vi "Get Total Plays.vi"(0 "File Directory":path, 11 "error in (no error)":errorcluster) -> (4 "Total Plays":i32, 15 "error out":errorcluster)   [LabVIEW 2014]
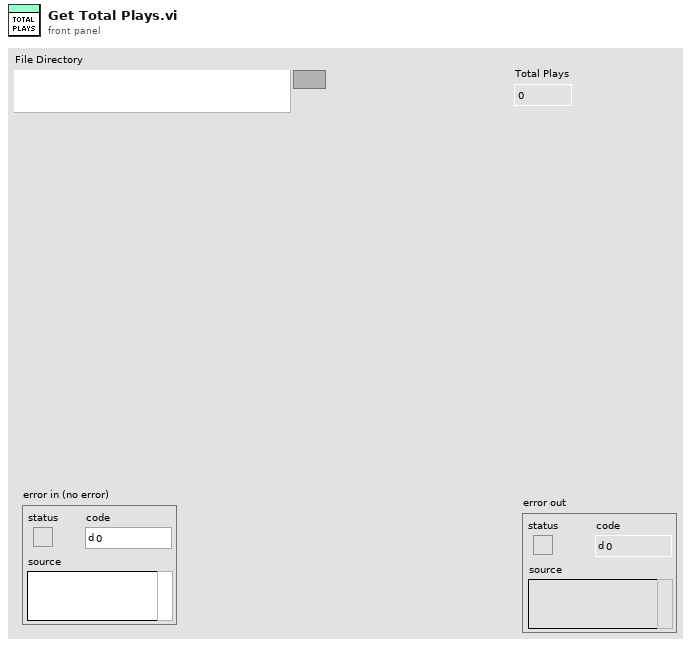
[diagram p1: front panel]
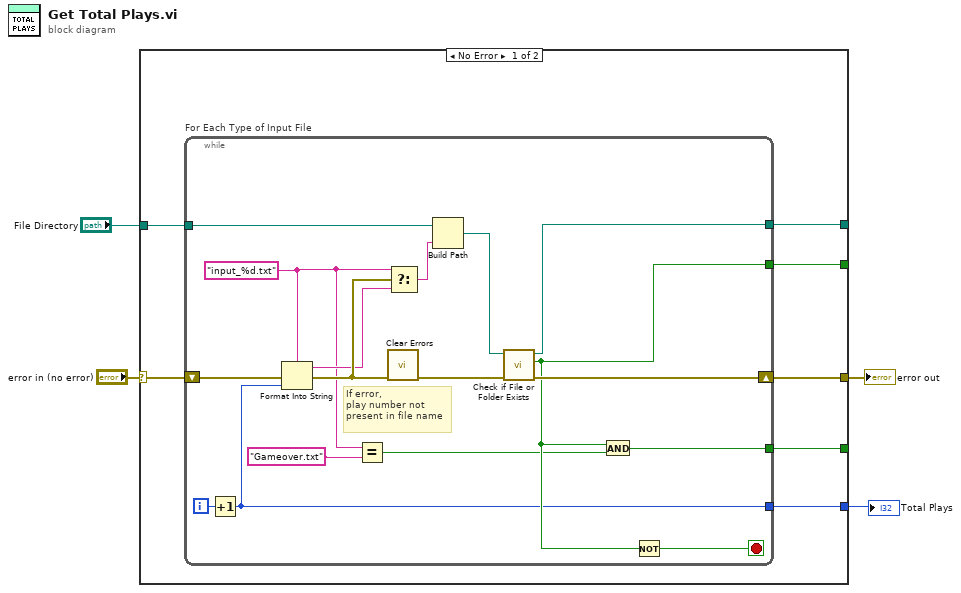
[diagram p0: block diagram]
diagram:
  n1 = case shown="No Error" "error in (no error)" {
    selector: "error in (no error)" -> [w11 w29]
    tunnel: "File Directory" -> [w10 _]
    tunnel: [w9 _] -> _
    tunnel: [w8 w29] -> w2
    tunnel: [w7 _] -> _
    tunnel: [w6 _] -> _
    tunnel: [w5 _] -> w1
    frame No Error {
      n2 = while "For Each Type of Input File" {
        tunnel: w10 -> [w22]
        shift-right: [w27] -> w8
        shift-left: w11 -> [w28]
        tunnel: [w26] -> w9
        tunnel: [w24] -> w7
        tunnel: [w23] -> w6
        tunnel: [w12] -> w5
        i -> [w13]
        stop <- w15 stop-if-true
        w14 = "input_%d.txt" ("String")
        # "If error,\nplay number not\npresent in file name"
        n3 = Increment(x=w13) -> (x+1=w12:i32)
        n4 = Format Into String(format string=w14, error in=w28, w12) -> (resulting string=w18:string, error out=w19:errorcluster)  [unwired: 1 in]
        n5 = Equal?(x=w14, y="Gameover.txt") -> (x = y?=w20:bool)
        n6 = call <vilib>:"Clear Errors.vi"("error in (no error)"=w19) -> ("error out"=w16:errorcluster)  [unwired: 5 in, 1 out]
        n7 = Select(t=w14, s=w19, f=w18) -> (s? t:f=w17:string)
        n8 = Build Path(base path=w22, name or relative path=w17) -> (appended path=w21:path)
        n9 = call <vilib>:"Check if File or Folder Exists.vi"("error in (no error)"=w16, "path"=w21) -> ("error out"=w27:errorcluster, "file or folder exists?"=w24:bool, "dup path"=w26:path)  [unwired: 7 in]
        n10 = And(x=w24, y=w20) -> (x .and. y?=w23:bool)
        n11 = Not(x=w24) -> (.not. x?=w15:bool)
      }
    }
    frame Error {
    }
  }
  "error out" <- w2
  "Total Plays" <- w1
